vi "rising edge.vi"(11 "APD1":bool) -> (3 "Boolean":bool)   [LabVIEW 2018, in "state machine.lvlib"]
uses:
  state machine.lvlib
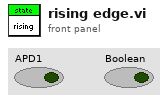
[diagram p1: front panel]
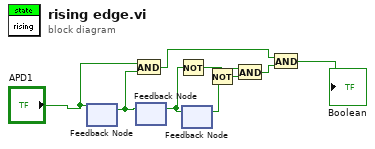
[diagram p0: block diagram]
diagram:
  n1 = feedback #1() -> (w1:bool)  [unwired: 1 in]
  n2 = feedback-in #1("APD1") -> ()
  n3 = And(x="APD1", y=w1) -> (x .and. y?=w8:bool)
  n4 = feedback #2() -> (w3:bool)  [unwired: 1 in]
  n5 = feedback-in #2(w1) -> ()
  n6 = Not(x=w3) -> (.not. x?=w5:bool)
  n7 = feedback #3() -> (w4:bool)  [unwired: 1 in]
  n8 = feedback-in #3(w3) -> ()
  n9 = Not(x=w4) -> (.not. x?=w6:bool)
  n10 = And(x=w5, y=w6) -> (x .and. y?=w7:bool)
  n11 = And(x=w8, y=w7) -> (x .and. y?=→"Boolean":bool)
